vi "CSMM6.contents.vi"   [LabVIEW 2012]
doc: "loads all VIs into memory required for building an application"
uses:
  MM6/MM6.lvlib
  MM6Archiver/MM6Archiver.lvlib
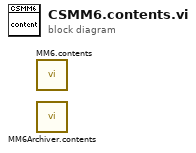
[diagram p0: block diagram]
diagram:
  n1 = call "MM6.contents.vi"() -> ()  [unwired: 1 in]
  n2 = call "MM6Archiver.contents.vi"() -> ()  [unwired: 1 in]
